vi "GoToSkill_v2.vi"(8 "error in (no error)":errorcluster, 10 "Robot":refnum<class "Robot.lvclass">, 11 "object in":refnum<class "GoToSkill_v2.lvclass">) -> (0 "error out":errorcluster, 2 "Robot out":refnum<class "Robot.lvclass">, 3 "object out":refnum<class "GoToSkill_v2.lvclass">)   [LabVIEW 2023, in "GoToSkill_v2.lvclass"]
uses:
  GoToSkill_v2.lvclass
  Robot_class/Robot.lvclass
  GoToSkill_v2.lvclass/GoToSkill_v2.ctl
  Robot_class/Robot.lvclass/Robot.ctl
  Robot_class/Write dest_x.vi
  Robot_class/Write dest_y.vi
  Robot_class/Write dest_orientation.vi
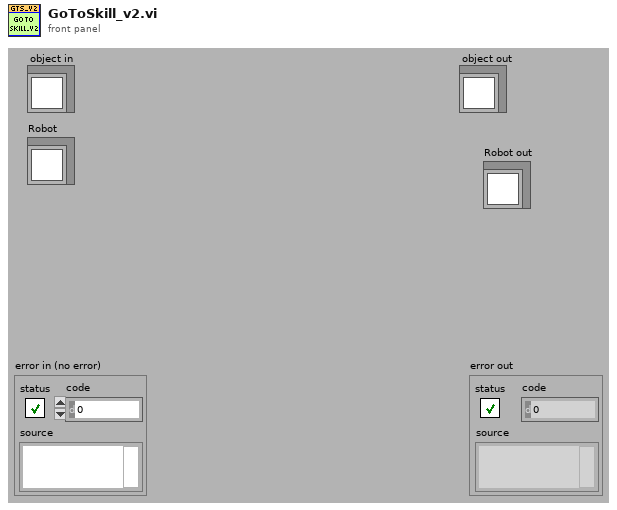
[diagram p1: front panel]
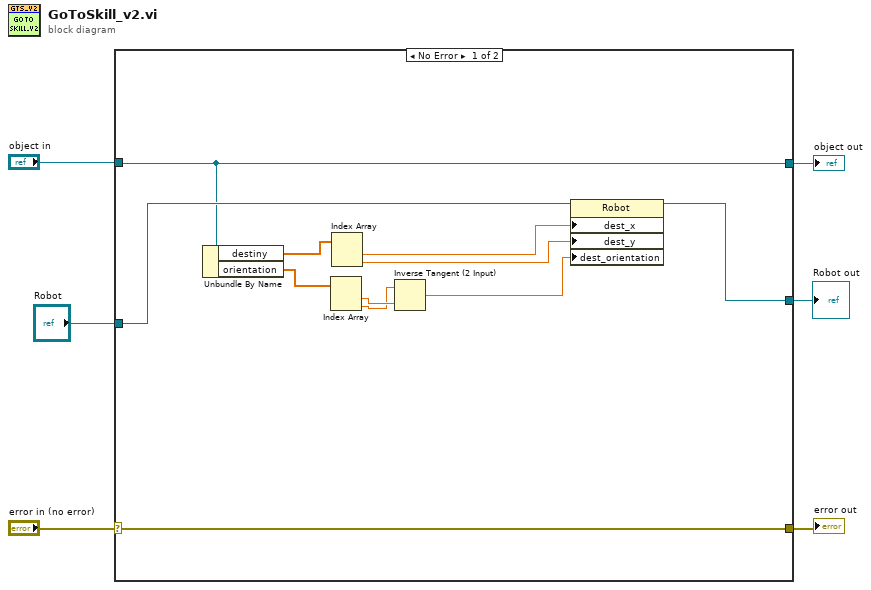
[diagram p0: block diagram]
diagram:
  n1 = case shown="No Error" "error in (no error)" {
    selector: "error in (no error)" -> [w17 w20]
    tunnel: [w17 w20] -> w5
    tunnel: [w14 w19] -> w3
    tunnel: "object in" -> [w14 w19]
    tunnel: [w16 w18] -> w2
    tunnel: "Robot" -> [w15 w18]
    frame No Error {
      n2 = Unbundle By Name(w14) -> ("destiny"=w12:dbl[], "orientation"=w13:dbl[])
      n3 = Index Array(array=w13) -> (element #1=w9:dbl, element #2=w8:dbl)  [unwired: 2 in]
      n4 = Index Array(array=w12) -> (element #1=w11:dbl, element #2=w10:dbl)  [unwired: 2 in]
      n5 = Inverse Tangent (2 Input)(1:w9, 2:w8) -> (0:w7:dbl)
      n6 = property class="Robot"(reference=w15, "dest_x"=w11, "dest_y"=w10, "dest_orientation"=w7) -> (reference out=w16:refnum<class "Robot.lvclass">)  [unwired: 1 in, 1 out]
    }
    frame Error {
    }
  }
  "error out" <- w5
  "object out" <- w3
  "Robot out" <- w2
